vi "Begin.vi"(8 "error in":errorcluster) -> (0 "error out":errorcluster)   [LabVIEW 2014]
doc: "Called before other user functions, this VI is expected to open initial I/O refnums, load in file data, and do all program initialization. Notice that the <B>error out</B> terminal is simply used for data flow. Wiring it to other structures or subVIs ensures that this VI runs first."
uses:
  <vilib>/Rock Robotics/WPI/DriverStation/WPI_DriverStationRobotMode2.ctl
  <vilib>/Rock Robotics/SystemInterfaces/DIO/FPGA_DIOChannel.ctl
  <vilib>/Rock Robotics/WPI/Encoder/WPI_EncoderType.ctl
  <vilib>/Rock Robotics/WPI/SPI/WPI_SPIMode.ctl
  <vilib>/Rock Robotics/SystemInterfaces/spilib/spi_bus.ctl
  <vilib>/Rock Robotics/WPI/CAN/TalonSRX/WPI_CANTalonSRX_APIControlMode.ctl
  <vilib>/Rock Robotics/WPI/Joystick/WPI_JoystickDeviceEnum.ctl
  <vilib>/Rock Robotics/WPI/SafetyOutput/WPI_SafetyOutputConfigMenu.ctl
  <vilib>/Rock Robotics/SystemInterfaces/AI/FPGA_AIChannel.ctl
  <vilib>/Rock Robotics/WPI/CAN/TalonSRX/WPI_CANTalonSRX_APIFeedbackSelect.ctl
  Robot Global Data.vi
  <vilib>/Rock Robotics/WPI/RobotDrive/WPI_RobotDriveOpen4MotorWithCANTalonSRX.vi
  <vilib>/Rock Robotics/WPI/Counter/WPI_CounterDigitalInputToDigitalSource.vi
  <vilib>/Rock Robotics/WPI/MotorControl/WPI_MotorControlOpenCANTalonSRX.vi
  <vilib>/Rock Robotics/WPI/Ultrasonic/WPI_SonarMB1010DigitalOpen.vi
  <vilib>/Rock Robotics/WPI/Ultrasonic/WPI_SonarMB1010DigRefNum Registry Set.vi
  <vilib>/Rock Robotics/WPI/Switch/WPI_SwitchOpenLimit.vi
panel:
  in  "PID gains 2":T1={"proportional gain (Kc)"=10.0, "integral time (Ti, min)"=0.0, "derivative time (Td, min)"=0.0} {"derivative time (Td, min)" format="%.3f"; "integral time (Ti, min)" format="%.3f"; "proportional gain (Kc)" format="%.3f"}
  in  "PID gains":T1={"proportional gain (Kc)"=1.0, "integral time (Ti, min)"=0.01, "derivative time (Td, min)"=0.0} {"derivative time (Td, min)" format="%.3f"; "integral time (Ti, min)" format="%.3f"; "proportional gain (Kc)" format="%.3f"}
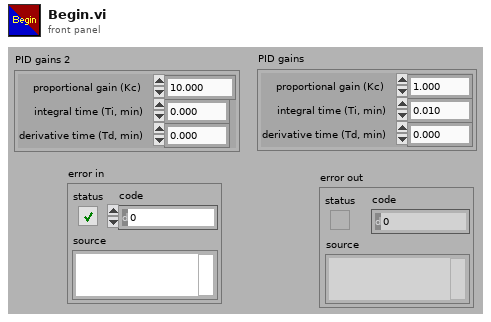
[diagram p1: front panel]
types:
  T1 = cluster{"proportional gain (Kc)":dbl, "integral time (Ti, min)":dbl, "derivative time (Td, min)":dbl}
  T2 = typedef "FPGA_DIOChannel.ctl" = enum8{"DIO 0", "DIO 1", "DIO 2", "DIO 3", "DIO 4", "DIO 5", "DIO 6", "DIO 7", "DIO 8", "DIO 9", "DIO MXP 0", "DIO MXP 1", "DIO MXP 2", "DIO MXP 3", "DIO MXP 4", "DIO MXP 5", "DIO MXP 6", "DIO MXP 7", "DIO MXP 8", "DIO MXP 9", "DIO MXP 10", "DIO MXP 11", "DIO MXP 12", "DIO MXP 13", "DIO MXP 14", "DIO MXP 15", "Invalid"}
  T3 = typedef "FPGA_AIChannel.ctl" = enum8{"AI 0", "AI 1", "AI 2", "AI 3", "AI MXP 0", "AI MXP 1", "AI MXP 2", "AI MXP 3", "Invalid"}
  T4 = typedef "WPI_SafetyOutputConfigMenu.ctl" = enum16{"Enable", "Disable"}
  T5 = typedef "WPI_CANTalonSRX_APIControlMode.ctl" = enum8{"Percent VBus", "Speed", "Position", "Slave", "Unchanged / Invalid"}
  T6 = typedef "WPI_JoystickDeviceEnum.ctl" = enum16{"USB 0", "USB 1", "USB 2", "USB 3", "USB 4", "USB 5"}
  T7 = typedef "spi_bus.ctl" = enum16{"SPI On-Board, CS0", "SPI On-Board, CS1", "SPI On-Board, CS2", "SPI On-Board, CS3", "SPI MXP", "Invalid"}
  T8 = typedef "WPI_SPIMode.ctl" = enum16{"Mode 0 (Clk Idle Low,Sample on Leading)", "Mode 1 (Clk Idle Low,Sample on Trailing)", "Mode 2 (Clk Idle High,Sample on Leading)", "Mode 3 (Clk Idle High,Sample on Trailing)"}
  T9 = typedef "WPI_EncoderType.ctl" = enum16{"1x", "2x", "4x"}
  T10 = typedef "WPI_DriverStationRobotMode2.ctl" = enum16{"Autonomous Disabled", "Autonomous Enabled", "Teleop Disabled", "Teleop Enabled", "Disconnected", "Finish", "Test Disabled", "Test Enabled", "Emergency Stopped"}
  T11 = typedef "WPI_CANTalonSRX_APIFeedbackSelect.ctl" = enum16{"Digital Quadrature Encoder", "Analog Potentiometer", "Analog Encoder"}
  T12 = typedef "WPI_MotorControlDeviceRef.ctl" = cluster{"DeviceStatus":errorcluster, "Type":T13, "PWM":cluster{"Controller":T14, "PWM Channel":T15, "DeadBand":T16}, "CAN":cluster{"Device Number":u8, "Control Mode":T17, "Semaphore":T18, "Max Vout":dbl, "TalonSRX Control Mode":T5}, "Invert":bool, "TransformRef":T19, "InvTransformRef":T19}
  T13 = typedef "WPI_MotorControlType.ctl" = enum16{"PWM", "CAN", "CANTalonSRX"}
  T14 = typedef "FPGA_TypedefDigitalModule.ctl" = enum16{"Controller 1"}
  T15 = typedef "FPGA_DIOPWMChannel.ctl" = enum8{"PWM 0", "PWM 1", "PWM 2", "PWM 3", "PWM 4", "PWM 5", "PWM 6", "PWM 7", "PWM 8", "PWM 9", "PWM MXP 0", "PWM MXP 1", "PWM MXP 2", "PWM MXP 3", "PWM MXP 4", "PWM MXP 5", "PWM MXP 6", "PWM MXP 7", "PWM MXP 8", "PWM MXP 9", "Invalid"}
  T16 = typedef "WPI_PWMDeadband.ctl" = cluster{"Name":string, "maxPositivePwm":i32, "minPositivePwm":i32, "centerPwm":i32, "maxNegativePwm":i32, "minNegativePwm":i32, "angularRange":u16}
  T17 = typedef "WPI_CANJaguar_ControlMode.ctl" = enum8{"Percent VBus", "Current", "Speed", "Position", "Voltage"}
  T18 = typedef "Semaphore RefNum" = refnum<k1>
  T19 = typedef "WPI_PWMTransform_ConPane.ctl" = refnum<vi>
  T20 = typedef "WPI_SwitchDevRef.ctl" = cluster{"DevStatus":errorcluster, "DIO Channel":T2, "Controller":T14, "CntIndex":T21, "Normally Closed":bool}
  T21 = typedef "FPGA_CounterCtrSystemIndex.ctl" = enum8{"Ctr 0", "Ctr 1", "Ctr 2", "Ctr 3", "Ctr 4", "Ctr 5", "Ctr 6", "Ctr 7", "Invalid"}
  T22 = typedef "WPI_PotentiometerDevRef.ctl" = cluster{"DevStatus":errorcluster, "Controller":T23, "Analog Channel":T3, "Invert Output":bool}
  T23 = typedef "FPGA_TypedefAnalogModule.ctl" = enum16{"Controller 1"}
  T24 = typedef "WPI_RobotDriveDevRef.ctl" = cluster{"DevStatus":errorcluster, "Motors[]":T12[], "Square Inputs":bool, "Max Output":dbl}
  T25 = typedef "WPI_JoystickDevRef.ctl" = cluster{"Device":T6}
  T26 = typedef "WPI_DigitalInputDevRef.ctl" = cluster{"DevStatus":errorcluster, "DIO Channel":T2, "Controller":T14}
  T27 = typedef "FPGA_CounterEncoderSourceConvertionLVSourceType.ctl" = cluster{"DevStatus":errorcluster, "AnalogTriggerMode?":bool, "DigitalMode":cluster{"Controller":T14, "DIO Channel":T28}, "AnalogTriggerMode":cluster{"AnalogTriggerIndex":T29, "OutputType":T30}}
  T28 = typedef "FPGA_DIODigitalSourceChannel.ctl" = enum8{"DIO 0", "DIO 1", "DIO 2", "DIO 3", "DIO 4", "DIO 5", "DIO 6", "DIO 7", "DIO 8", "DIO 9", "DIO MXP 0", "DIO MXP 1", "DIO MXP 2", "DIO MXP 3", "DIO MXP 4", "DIO MXP 5", "DIO MXP 6", "DIO MXP 7", "DIO MXP 8", "DIO MXP 9", "DIO MXP 10", "DIO MXP 11", "DIO MXP 12", "DIO MXP 13", "DIO MXP 14", "DIO MXP 15", "Disabled"}
  T29 = typedef "FPGA_AnalogTriggerIndex.ctl" = enum8{"Trig 0", "Trig 1", "Trig 2", "Trig 3", "Trig 4", "Trig 5", "Trig 6", "Trig 7", "Invalid"}
  T30 = typedef "FPGA_AnalogTriggerOutType.ctl" = enum16{"InWindow", "TriggerState", "Rising", "Falling"}
  T31 = typedef "WPI_SonarMB1010DigitalDeviceRef.ctl" = cluster{"CounterDevRef":T32, "Scaling factor (s/in)":dbl}
  T32 = typedef "WPI_CounterDevRef.ctl" = cluster{"DevStatus":errorcluster, "CntIndex":T21}
  T33 = typedef "WPI_SPIDevRef.ctl" = cluster{"DevStatus":errorcluster, "Handle":i32, "Controller":T14, "SPI Bus":T7}
  T34 = typedef "WPI_EncoderDevRef.ctl" = cluster{"DevStatus":errorcluster, "EncoderIndex":T35, "CounterIndex":T21, "DistancePerCount":dbl, "Decoding Type":T9}
  T35 = typedef "FPGA_EncoderIdx.ctl" = enum8{"Enc 0", "Enc 1", "Enc 2", "Enc 3", "Enc 4", "Enc 5", "Enc 6", "Enc 7", "Invalid"}
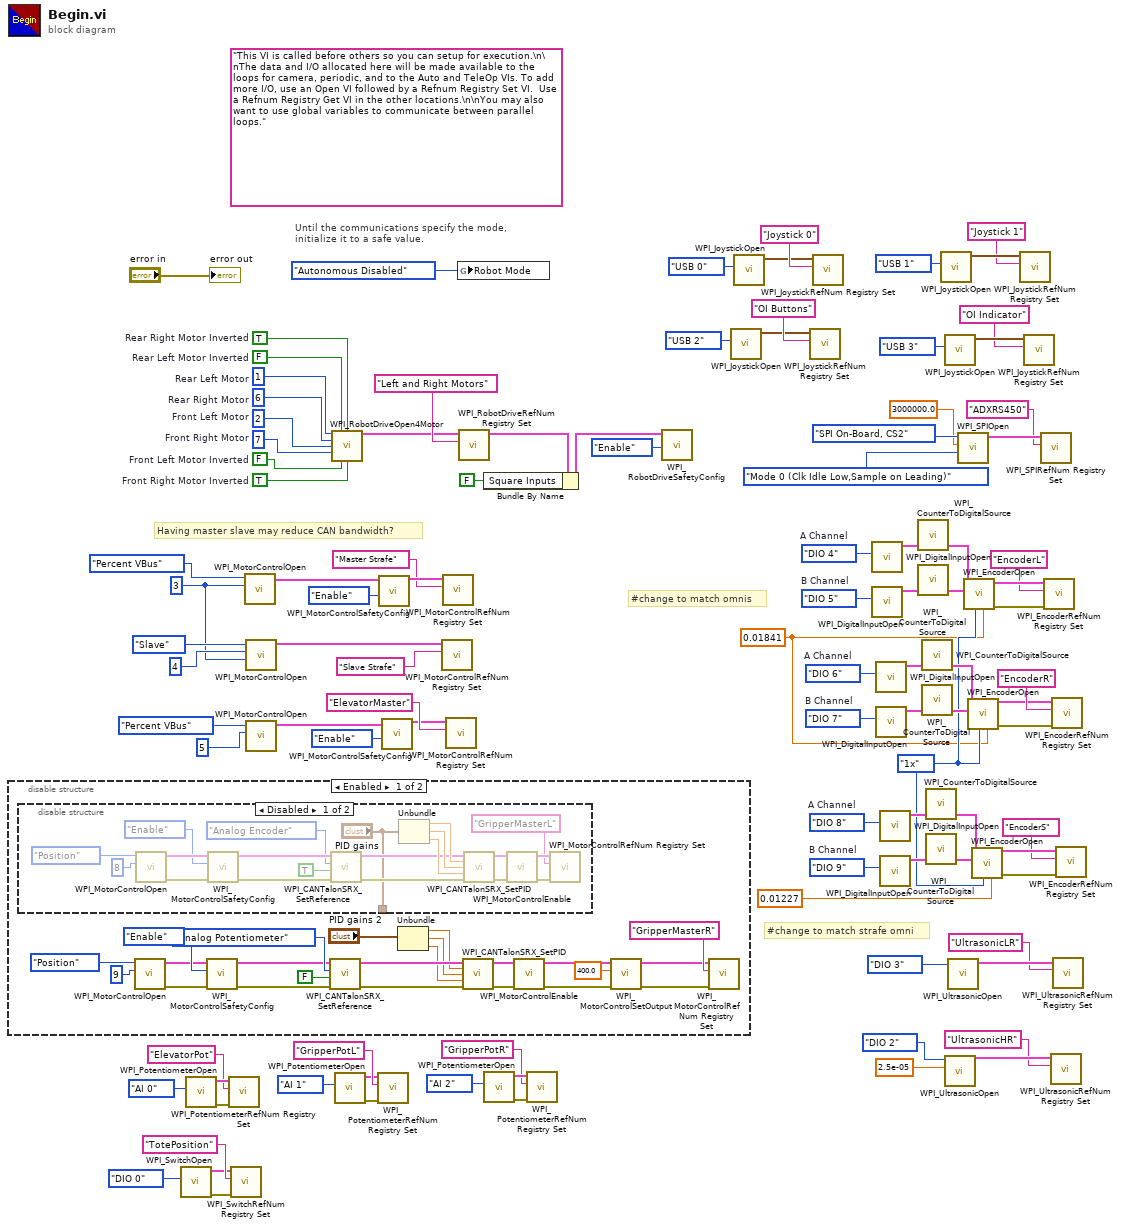
[diagram p0: block diagram]
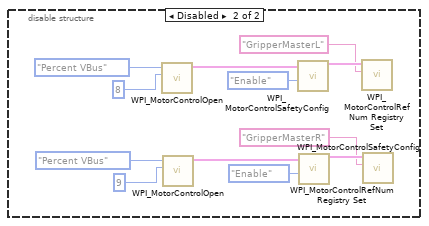
[diagram p3: hidden frame]
diagram:
  w48 = u8 3 ("Device Number")
  w60 = FPGA_DIOChannel."DIO 9"  # B Channel
  w59 = FPGA_DIOChannel."DIO 8"  # A Channel
  w54 = WPI_EncoderType."1x" ("Decoding Type")
  w53 = 0.01841 ("DistancePerCount")
  w76 = FPGA_DIOChannel."DIO 7"  # B Channel
  w77 = FPGA_DIOChannel."DIO 6"  # A Channel
  w87 = FPGA_DIOChannel."DIO 5"  # B Channel
  w86 = FPGA_DIOChannel."DIO 4"  # A Channel
  w88 = TRUE  # Rear Right Motor Inverted
  w89 = FALSE  # Rear Left Motor Inverted
  w90 = TRUE  # Front Right Motor Inverted
  w91 = FALSE  # Front Left Motor Inverted
  w92 = u8 7  # Front Right Motor
  w93 = u8 2  # Front Left Motor
  w94 = u8 6  # Rear Right Motor
  w95 = u8 1  # Rear Left Motor
  (unwired) "This VI is called before others so you can setup for execution.\n\nThe data and I/O allocated here will be made available to the loops for camera, periodic, and to the Auto and TeleOp VIs. To add more I/O, use an Open VI followed by a Refnum Registry Set VI.  Use a Refnum Registry Get VI in the other locations.\n\nYou may also want to use global variables to communicate between parallel loops."
  # "Having master slave may reduce CAN bandwidth?"
  # "#change to match strafe omni"
  # "#change to match omnis"
  # "Until the communications specify the mode,\ninitialize it to a safe value."
  n1 = disable-structure shown="Enabled" {
    frame Enabled {
      n2 = disable-structure shown="Disabled" {
        disable-tunnel: ["PID gains" _] -> _
        frame Disabled {
          n3 = call-poly <vilib>:"WPI_MotorControlOpen.vi"("Device Number"=u8 8, "Control Mode"=WPI_CANTalonSRX_APIControlMode."Position") -> ("error out"=w143:errorcluster, "MotorControlDeviceRef"=w131:T12)  [unwired: 8 in]
          n4 = call <vilib>:"WPI_MotorControlSafetyConfig.vi"("error in (no error)"=w143, "mode"=WPI_SafetyOutputConfigMenu."Enable", "MotorControlDevRef"=w131) -> ("error out"=w145:errorcluster, "MotorControlDevRef"=w144:T12)  [unwired: 7 in]
          n5 = call <vilib>:"WPI_CANTalonSRX_SetReference.vi"("error in (no error)"=w145, "Reverse Feedback Sensor"=TRUE, "Feedback Reference"=WPI_CANTalonSRX_APIFeedbackSelect."Analog Encoder", "CAN Talon SRX Ref"=w144) -> ("error out"=w137:errorcluster, "CAN Talon SRX Ref Out"=w132:T12)  [unwired: 6 in]
          n6 = Unbundle("PID gains") -> ("proportional gain (Kc)"=w140:dbl, "integral time (Ti, min)"=w141:dbl, "derivative time (Td, min)"=w142:dbl)
          n7 = call <vilib>:"WPI_CANTalonSRX_SetPID.vi"("CAN Talon SRX Ref"=w132, "P"=w140, "I"=w141, "D"=w142, "error in (no error)"=w137) -> ("CAN Talon SRX Ref Out"=w133:T12, "error out"=w134:errorcluster)  [unwired: 9 in]
          n8 = call <vilib>:"WPI_MotorControlEnable.vi"("error in (no error)"=w134, "CAN Jaguar Ref"=w133) -> ("error out"=w136:errorcluster, "CAN Jaguar Ref Out"=w135:T12)  [unwired: 8 in]
          n9 = call <vilib>:"WPI_MotorControlRefNum Registry Set.vi"("error in (no error)"=w136, "refnum name"="GripperMasterL", "MotorControlDevRef"=w135) -> ()  [unwired: 7 in, 2 out]
        }
        frame Enabled {
        }
      }
      n10 = call-poly <vilib>:"WPI_MotorControlOpen.vi"("Device Number"=u8 9, "Control Mode"=WPI_CANTalonSRX_APIControlMode."Position") -> ("error out"=w110:errorcluster, "MotorControlDeviceRef"=w121:T12)  [unwired: 8 in]
      n11 = call <vilib>:"WPI_MotorControlSafetyConfig.vi"("error in (no error)"=w110, "mode"=WPI_SafetyOutputConfigMenu."Enable", "MotorControlDevRef"=w121) -> ("error out"=w108:errorcluster, "MotorControlDevRef"=w109:T12)  [unwired: 7 in]
      n12 = call <vilib>:"WPI_CANTalonSRX_SetReference.vi"("error in (no error)"=w108, "Reverse Feedback Sensor"=FALSE, "Feedback Reference"=WPI_CANTalonSRX_APIFeedbackSelect."Analog Potentiometer", "CAN Talon SRX Ref"=w109) -> ("error out"=w116:errorcluster, "CAN Talon SRX Ref Out"=w120:T12)  [unwired: 6 in]
      n13 = Unbundle("PID gains 2") -> ("proportional gain (Kc)"=w113:dbl, "integral time (Ti, min)"=w112:dbl, "derivative time (Td, min)"=w111:dbl)
      n14 = call <vilib>:"WPI_CANTalonSRX_SetPID.vi"("CAN Talon SRX Ref"=w120, "P"=w113, "I"=w112, "D"=w111, "error in (no error)"=w116) -> ("CAN Talon SRX Ref Out"=w119:T12, "error out"=w118:errorcluster)  [unwired: 9 in]
      n15 = call <vilib>:"WPI_MotorControlEnable.vi"("error in (no error)"=w118, "CAN Jaguar Ref"=w119) -> ("error out"=w117:errorcluster, "CAN Jaguar Ref Out"=w105:T12)  [unwired: 8 in]
      n16 = call <vilib>:"WPI_MotorControlSetOutput.vi"("error in (no error)"=w117, "Output"=400.0, "MotorControlDevRef"=w105) -> ("error out"=w106:errorcluster, "MotorControlDevRef"=w104:T12)  [unwired: 6 in, 1 out]
      n17 = call <vilib>:"WPI_MotorControlRefNum Registry Set.vi"("error in (no error)"=w106, "refnum name"="GripperMasterR", "MotorControlDevRef"=w104) -> ()  [unwired: 7 in, 2 out]
    }
    frame Disabled {
      n18 = call-poly <vilib>:"WPI_MotorControlOpen.vi"("Device Number"=u8 8, "Control Mode"=WPI_CANTalonSRX_APIControlMode."Percent VBus") -> ("MotorControlDeviceRef"=w153:T12)  [unwired: 8 in, 1 out]
      n19 = call-poly <vilib>:"WPI_MotorControlOpen.vi"("Device Number"=u8 9, "Control Mode"=WPI_CANTalonSRX_APIControlMode."Percent VBus") -> ("MotorControlDeviceRef"=w152:T12)  [unwired: 8 in, 1 out]
      n20 = call <vilib>:"WPI_MotorControlSafetyConfig.vi"("mode"=WPI_SafetyOutputConfigMenu."Enable", "MotorControlDevRef"=w153) -> ("MotorControlDevRef"=w155:T12)  [unwired: 8 in, 1 out]
      n21 = call <vilib>:"WPI_MotorControlSafetyConfig.vi"("mode"=WPI_SafetyOutputConfigMenu."Enable", "MotorControlDevRef"=w152) -> ("MotorControlDevRef"=w150:T12)  [unwired: 8 in, 1 out]
      n22 = call <vilib>:"WPI_MotorControlRefNum Registry Set.vi"("refnum name"="GripperMasterL", "MotorControlDevRef"=w155) -> ()  [unwired: 8 in, 2 out]
      n23 = call <vilib>:"WPI_MotorControlRefNum Registry Set.vi"("refnum name"="GripperMasterR", "MotorControlDevRef"=w150) -> ()  [unwired: 8 in, 2 out]
    }
  }
  n24 = call-poly <vilib>:"WPI_SwitchOpen.vi"("DIO Channel"=FPGA_DIOChannel."DIO 0") -> ("error out"=w1:errorcluster, "SwitchDevRef"=w2:T20)  [unwired: 9 in]
  n25 = call <vilib>:"WPI_PotentiometerOpen.vi"("Analog Channel"=FPGA_AIChannel."AI 0") -> ("error out"=w20:errorcluster, "PotDevRef"=w23:T22)  [unwired: 9 in]
  n26 = call <vilib>:"WPI_PotentiometerRefNum Registry Set.vi"("error in (no error)"=w20, "refnum name"="ElevatorPot", "PotDevRef"=w23) -> ()  [unwired: 7 in, 2 out]
  n27 = call <vilib>:"WPI_SwitchRefNum Registry Set.vi"("error in (no error)"=w1, "refnum name"="TotePosition", "SwitchDevRef"=w2) -> ()  [unwired: 7 in, 2 out]
  n28 = call-poly <vilib>:"WPI_MotorControlOpen.vi"("Device Number"=w48, "Control Mode"=WPI_CANTalonSRX_APIControlMode."Percent VBus") -> ("MotorControlDeviceRef"=w46:T12)  [unwired: 8 in, 1 out]
  n29 = call-poly <vilib>:"WPI_MotorControlOpen.vi"("Master Device Number"=w48, "Device Number"=u8 4, "Control Mode"=WPI_CANTalonSRX_APIControlMode."Slave") -> ("MotorControlDeviceRef"=w43:T12)  [unwired: 7 in, 1 out]
  n30 = call-poly <vilib>:"WPI_MotorControlOpen.vi"("Device Number"=u8 5, "Control Mode"=WPI_CANTalonSRX_APIControlMode."Percent VBus") -> ("MotorControlDeviceRef"=w24:T12)  [unwired: 8 in, 1 out]
  n31 = call-poly <vilib>:"WPI_RobotDriveOpen4Motor.vi"("Rear Left Motor"=w95, "Rear Left Motor Inverted"=w89, "Rear Right Motor Inverted"=w88, "Rear Right Motor"=w94, "Front Left Motor"=w93, "Front Right Motor"=w92, "Front Left Motor Inverted"=w91, "Front Right Motor Inverted"=w90) -> ("RobotDriveDevRef"=w64:T24)  [unwired: 6 in, 1 out]
  n32 = call <vilib>:"WPI_PotentiometerOpen.vi"("Analog Channel"=FPGA_AIChannel."AI 1") -> ("error out"=w19:errorcluster, "PotDevRef"=w16:T22)  [unwired: 9 in]
  n33 = call <vilib>:"WPI_PotentiometerRefNum Registry Set.vi"("error in (no error)"=w19, "refnum name"="GripperPotL", "PotDevRef"=w16) -> ()  [unwired: 7 in, 2 out]
  n34 = call <vilib>:"WPI_MotorControlSafetyConfig.vi"("mode"=WPI_SafetyOutputConfigMenu."Enable", "MotorControlDevRef"=w46) -> ("MotorControlDevRef"=w45:T12)  [unwired: 8 in, 1 out]
  n35 = call <vilib>:"WPI_MotorControlSafetyConfig.vi"("mode"=WPI_SafetyOutputConfigMenu."Enable", "MotorControlDevRef"=w24) -> ("MotorControlDevRef"=w26:T12)  [unwired: 8 in, 1 out]
  n36 = call <vilib>:"WPI_MotorControlRefNum Registry Set.vi"("refnum name"="Slave Strafe", "MotorControlDevRef"=w43) -> ()  [unwired: 8 in, 2 out]
  n37 = call <vilib>:"WPI_MotorControlRefNum Registry Set.vi"("refnum name"="Master Strafe", "MotorControlDevRef"=w45) -> ()  [unwired: 8 in, 2 out]
  n38 = call <vilib>:"WPI_MotorControlRefNum Registry Set.vi"("refnum name"="ElevatorMaster", "MotorControlDevRef"=w26) -> ()  [unwired: 8 in, 2 out]
  n39 = global write "Robot Global Data.vi" "Robot Mode"(WPI_DriverStationRobotMode2."Autonomous Disabled" ("Robot Mode")) -> ()
  n40 = call <vilib>:"WPI_RobotDriveRefNum Registry Set.vi"("refnum name"="Left and Right Motors", "RobotDriveDevRef"=w64) -> ("RobotDriveDevRef"=w98:T24)  [unwired: 1 in, 8 out]
  n41 = Bundle By Name(cluster=w98, "Square Inputs"=FALSE) -> (w97:T24)
  n42 = call <vilib>:"WPI_PotentiometerOpen.vi"("Analog Channel"=FPGA_AIChannel."AI 2") -> ("error out"=w12:errorcluster, "PotDevRef"=w15:T22)  [unwired: 9 in]
  n43 = call <vilib>:"WPI_PotentiometerRefNum Registry Set.vi"("error in (no error)"=w12, "refnum name"="GripperPotR", "PotDevRef"=w15) -> ()  [unwired: 7 in, 2 out]
  n44 = call <vilib>:"WPI_RobotDriveSafetyConfig.vi"("mode"=WPI_SafetyOutputConfigMenu."Enable", "RobotDriveDevRef"=w97) -> ()  [unwired: 8 in, 2 out]
  n45 = call <vilib>:"WPI_JoystickOpen.vi"("JoystickDevice"=WPI_JoystickDeviceEnum."USB 2") -> ("JoystickDevRef"=w34:T25)  [unwired: 10 in]
  n46 = call <vilib>:"WPI_JoystickOpen.vi"("JoystickDevice"=WPI_JoystickDeviceEnum."USB 0") -> ("JoystickDevRef"=w40:T25)  [unwired: 10 in]
  n47 = call <vilib>:"WPI_JoystickRefNum Registry Set.vi"("refnum name"="OI Buttons", "JoystickDevRef"=w34) -> ()  [unwired: 8 in, 2 out]
  n48 = call <vilib>:"WPI_JoystickRefNum Registry Set.vi"("refnum name"="Joystick 0", "JoystickDevRef"=w40) -> ()  [unwired: 8 in, 2 out]
  n49 = call <vilib>:"WPI_DigitalInputOpen.vi"("DIO Channel"=w86) -> ("DigitalInputDevRef"=w83:T26)  [unwired: 2 in, 8 out]
  n50 = call <vilib>:"WPI_DigitalInputOpen.vi"("DIO Channel"=w87) -> ("DigitalInputDevRef"=w84:T26)  [unwired: 2 in, 8 out]
  n51 = call <vilib>:"WPI_DigitalInputOpen.vi"("DIO Channel"=w77) -> ("DigitalInputDevRef"=w80:T26)  [unwired: 2 in, 8 out]
  n52 = call <vilib>:"WPI_DigitalInputOpen.vi"("DIO Channel"=w76) -> ("DigitalInputDevRef"=w79:T26)  [unwired: 2 in, 8 out]
  n53 = call <vilib>:"WPI_DigitalInputOpen.vi"("DIO Channel"=w59) -> ("DigitalInputDevRef"=w56:T26)  [unwired: 2 in, 8 out]
  n54 = call <vilib>:"WPI_DigitalInputOpen.vi"("DIO Channel"=w60) -> ("DigitalInputDevRef"=w57:T26)  [unwired: 2 in, 8 out]
  n55 = call-poly <vilib>:"WPI_CounterToDigitalSource.vi"("DigitalInputDevRef"=w83) -> ("Digital Source"=w82:T27)  [unwired: 6 out]
  n56 = call-poly <vilib>:"WPI_CounterToDigitalSource.vi"("DigitalInputDevRef"=w84) -> ("Digital Source"=w85:T27)  [unwired: 6 out]
  n57 = call-poly <vilib>:"WPI_CounterToDigitalSource.vi"("DigitalInputDevRef"=w80) -> ("Digital Source"=w81:T27)  [unwired: 6 out]
  n58 = call-poly <vilib>:"WPI_CounterToDigitalSource.vi"("DigitalInputDevRef"=w79) -> ("Digital Source"=w78:T27)  [unwired: 6 out]
  n59 = call-poly <vilib>:"WPI_CounterToDigitalSource.vi"("DigitalInputDevRef"=w56) -> ("Digital Source"=w55:T27)  [unwired: 6 out]
  n60 = call-poly <vilib>:"WPI_CounterToDigitalSource.vi"("DigitalInputDevRef"=w57) -> ("Digital Source"=w58:T27)  [unwired: 6 out]
  n61 = call <vilib>:"WPI_JoystickOpen.vi"("JoystickDevice"=WPI_JoystickDeviceEnum."USB 1") -> ("JoystickDevRef"=w37:T25)  [unwired: 10 in]
  n62 = call <vilib>:"WPI_JoystickOpen.vi"("JoystickDevice"=WPI_JoystickDeviceEnum."USB 3") -> ("JoystickDevRef"=w31:T25)  [unwired: 10 in]
  n63 = call-poly <vilib>:"WPI_UltrasonicOpen.vi"("Scaling factor (s/in)"=2.5e-05, "DIO Channel"=FPGA_DIOChannel."DIO 2") -> ("SonarMB1010DigitalDevRef"=w10:T31)  [unwired: 8 in, 1 out]
  n64 = call-poly <vilib>:"WPI_UltrasonicOpen.vi"("DIO Channel"=FPGA_DIOChannel."DIO 3") -> ("SonarMB1010DigitalDevRef"=w11:T31)  [unwired: 9 in, 1 out]
  n65 = call <vilib>:"WPI_SPIOpen.vi"("Mode (3)"=WPI_SPIMode."Mode 0 (Clk Idle Low,Sample on Leading)", "Clock Rate (Hz)"=3000000.0, "SPI Bus"=spi_bus."SPI On-Board, CS2") -> ("SPIDevRef"=w66:T33)  [unwired: 3 in, 5 out]
  n66 = call <vilib>:"WPI_EncoderOpen.vi"("DistancePerCount"=w53, "Decoding Type"=w54, "BSource"=w85, "ASource"=w82) -> ("error out"=w74:errorcluster, "EncoderDevRef"=w75:T34)  [unwired: 4 in, 2 out]
  n67 = call <vilib>:"WPI_EncoderOpen.vi"("DistancePerCount"=w53, "Decoding Type"=w54, "BSource"=w78, "ASource"=w81) -> ("error out"=w70:errorcluster, "EncoderDevRef"=w71:T34)  [unwired: 4 in, 2 out]
  n68 = call <vilib>:"WPI_EncoderOpen.vi"("DistancePerCount"=0.01227, "Decoding Type"=w54, "BSource"=w58, "ASource"=w55) -> ("error out"=w63:errorcluster, "EncoderDevRef"=w62:T34)  [unwired: 4 in, 2 out]
  n69 = call <vilib>:"WPI_JoystickRefNum Registry Set.vi"("refnum name"="Joystick 1", "JoystickDevRef"=w37) -> ()  [unwired: 8 in, 2 out]
  n70 = call <vilib>:"WPI_JoystickRefNum Registry Set.vi"("refnum name"="OI Indicator", "JoystickDevRef"=w31) -> ()  [unwired: 8 in, 2 out]
  n71 = call <vilib>:"WPI_SPIRefNum Registry Set.vi"("refnum name"="ADXRS450", "SPIDevRef"=w66) -> ()  [unwired: 8 in, 2 out]
  n72 = call <vilib>:"WPI_EncoderRefNum Registry Set.vi"("error in (no error)"=w74, "refnum name"="EncoderL", "EncoderDevRef"=w75) -> ()  [unwired: 7 in, 2 out]
  n73 = call-poly <vilib>:"WPI_UltrasonicRefNum Registry Set.vi"("refnum name"="UltrasonicHR", "SonarMB1010DigitalDevRef"=w10) -> ()  [unwired: 8 in, 2 out]
  n74 = call <vilib>:"WPI_EncoderRefNum Registry Set.vi"("error in (no error)"=w70, "refnum name"="EncoderR", "EncoderDevRef"=w71) -> ()  [unwired: 7 in, 2 out]
  n75 = call-poly <vilib>:"WPI_UltrasonicRefNum Registry Set.vi"("refnum name"="UltrasonicLR", "SonarMB1010DigitalDevRef"=w11) -> ()  [unwired: 8 in, 2 out]
  n76 = call <vilib>:"WPI_EncoderRefNum Registry Set.vi"("error in (no error)"=w63, "refnum name"="EncoderS", "EncoderDevRef"=w62) -> ()  [unwired: 7 in, 2 out]
  "error out" <- "error in"
